vi "WS2812 Write One Pixel.vi"(7 "Refresh? (T)":bool=TRUE, 8 "Error In":errorcluster, 9 "Color":u32(colorbox), 10 "Pixel Index":u16, 11 "LINX Device Config":T1) -> (0 "Error Out":errorcluster, 3 "LINX Device Config":T1)   [LabVIEW 2020, in "LMH-LINX.lvlib" / "Device.lvlib"]
uses:
  Device.lvlib
  Type Defs/LINX Device Config.ctl
  Type Defs/Interface.ctl
  Type Defs/TCP Config.ctl
  Type Defs/Channels.ctl
  Type Defs/Error Type.ctl
  LMH-LINX.lvlib
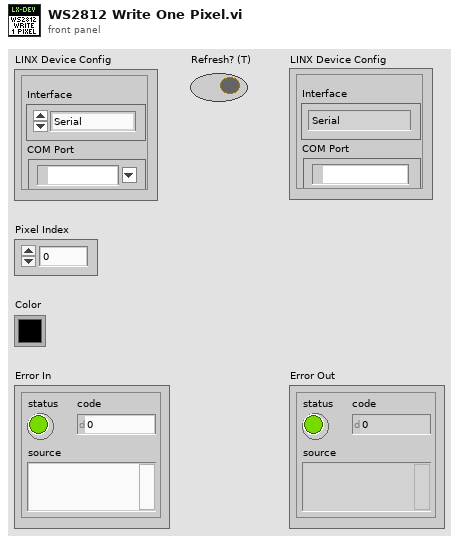
[diagram p1: front panel]
types:
  T1 = typedef "LMH-LINX.lvlib/Device.lvlib/LINX Device Config.ctl" = cluster{"Interface":T2, "COM Port":refnum<visa-resource-name>, "TCP Configuration":T3, "Device Family":u8, "Device ID":u8, "Device Name":string, "TCP Ref":refnum<k5>, "Channels":T4}
  T2 = typedef "LMH-LINX.lvlib/Interface.ctl" = enum16{"Serial", "TCP"}
  T3 = typedef "LMH-LINX.lvlib/Device.lvlib/TCP Config.ctl" = cluster{"IP Address":string, "Port":u16}
  T4 = typedef "LMH-LINX.lvlib/Channels.ctl" = cluster{"DI":u8[], "DO":u8[], "AI":u8[], "AO":u8[], "PWM":u8[], "QE":u8[], "UART":u8[], "I2C 2":u8[], "SPI":u8[], "CAN":u8[], "Servo":u8[], "AI Ref (V)":dbl, "AI Resolution (Bits)":u8, "AO Ref (V)":dbl, "AO Resolution (Bits)":u8}
  T5 = typedef "LMH-LINX.lvlib/Error Type.ctl" = enum16{"Unknown", "Timeout", "Corrupt Return Packet", "Unable To Connect", "Command Not Supported", "Channel DNE", "Invalid COM Config", "Firmware Version Mismatch", "myRIO Support", "CMD Specific Error", "Local IO Not Supported"}
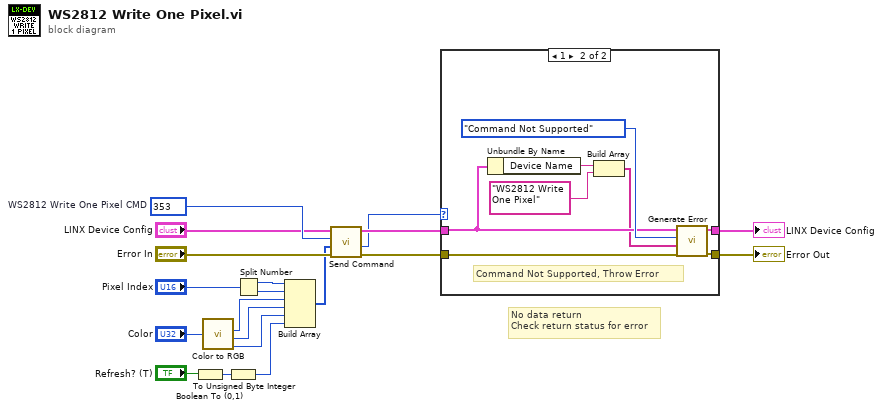
[diagram p0: block diagram]
diagram:
  w19 = u16 353  # WS2812 Write One Pixel CMD
  # "No data return\nCheck return status for error"
  n1 = Boolean To (0,1)(Boolean="Refresh? (T)") -> (0, 1=w6:i16)
  n2 = call <vilib>:"Color to RGB.vi"("Color"="Color") -> ("R"=w4:u8, "G"=w3:u8, "B"=w2:u8)  [unwired: 1 out]
  n3 = To Unsigned Byte Integer(number=w6) -> (unsigned 8bit integer=w5:u8)
  n4 = Split Number(x="Pixel Index") -> (hi(x)=w10:u8, lo(x)=w9:u8)
  n5 = Build Array(w10, w9, w4, w3, w2, w5) -> (w8:u8[])
  n6 = call "Send Command.vi"("Error In"="Error In", "ARGS"=w8, "CMD"=w19, "LINX Device Config"="LINX Device Config") -> ("Error Out"=w16:errorcluster, "Status"=w14:u8, "LINX Device Config"=w15:T1)  [unwired: 4 in, 1 out]
  n7 = case shown="1" w14 {
    tunnel: [w21 w27] -> w18
    tunnel: w15 -> [w21 w23]
    tunnel: [w20 w28] -> w17
    tunnel: w16 -> [w20 w29]
    frame 0, Default {
      # "Status OK"
    }
    frame 1 {
      # "Command Not Supported, Throw Error"
      n8 = Unbundle By Name(w23) -> ("Device Name"=w25:string)
      n9 = Build Array(w25, "WS2812 Write One Pixel") -> (w22:string[])
      n10 = call "Generate Error.vi"("Error In"=w29, "Arguments"=w22, "Error Type"=Error_Type."Command Not Supported", "LINX Device Config"=w23) -> ("Error Out"=w28:errorcluster, "Dup LINX Device Config"=w27:T1)  [unwired: 6 in]
    }
  }
  "Error Out" <- w17
  "LINX Device Config" <- w18
